vi "move_andor_files.vi"(8 "error in":errorcluster, 10 "Data Files Path":path, 11 "Andor setup":T1) -> (0 "error out":errorcluster)   [LabVIEW 2013]
uses:
  Andor_settings.ctl
  Globals.vi
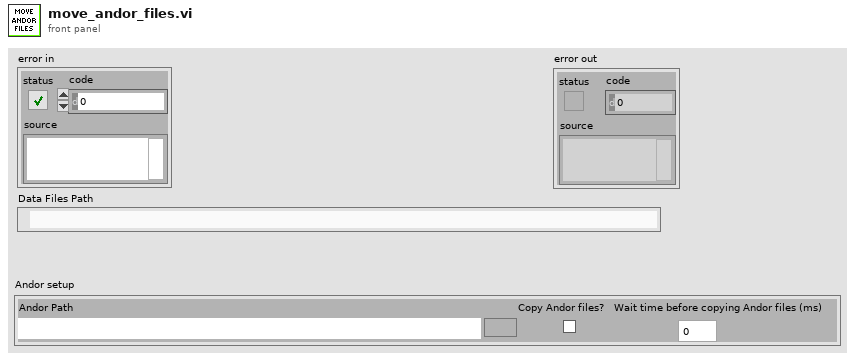
[diagram p1: front panel]
types:
  T1 = typedef "Andor_settings.ctl" = cluster{"Andor Path":path, "Copy any Andor files":bool, "Wait time before copying Andor files (ms)":u16}
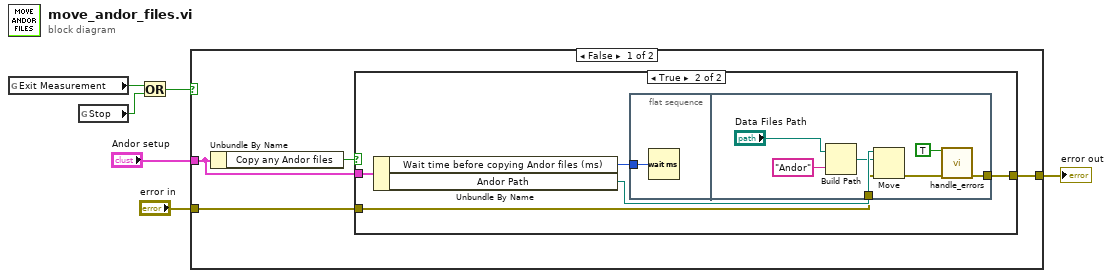
[diagram p0: block diagram]
diagram:
  n1 = global read "Globals.vi" "Exit Measurement"() -> (w3:bool)
  n2 = global read "Globals.vi" "Stop"() -> (w2:bool)
  n3 = Or(x=w3, y=w2) -> (x .or. y?=w1:bool)
  n4 = case shown="False" w1 {
    tunnel: "Andor setup" -> [w9 _]
    tunnel: "error in" -> [w8 w26]
    tunnel: [w7 w26] -> w4
    frame False {
      n5 = Unbundle By Name(w9) -> ("Copy any Andor files"=w10:bool)
      n6 = case shown="True" w10 {
        tunnel: w9 -> [_ w16]
        tunnel: w8 -> [w11 w13]
        tunnel: [w11 w12] -> w7
        frame False {
        }
        frame True {
          n7 = Unbundle By Name(w16) -> ("Wait time before copying Andor files (ms)"=w15:u16, "Andor Path"=w14:path)
          n8 = flat-sequence {
            tunnel: w15 -> [w17]
            tunnel: w14 -> [w25]
            tunnel: w13 -> [w23]
            tunnel: [w22] -> w12
            frame #0 {
              n9 = Wait (ms)(milliseconds to wait=w17) -> ()  [unwired: 1 out]
            }
            frame #1 {
              n10 = Build Path(base path="Data Files Path", name or relative path="Andor") -> (appended path=w19:path)
              n11 = Move(source path=w25, error in=w23, 10:w19) -> (error out=w24:errorcluster)  [unwired: 2 in, 2 out]
              n12 = call "handle_errors.vi"("Exit Operation"=TRUE ("Exit Measurement"), "error in (no error)"=w24) -> ("error out"=w22:errorcluster)  [unwired: 13 in]
            }
          }
        }
      }
    }
    frame True {
    }
  }
  "error out" <- w4
